vi "Array_extraction(SubVI).vi"(11 "Array":dbl[](array[numeric])) -> (1 "Value":dbl, 2 "Iteration":dbl, 3 "Info":dbl)   [LabVIEW 2017]
doc: "SubVI that extracts values from <B>Array</B> into three double values.\n<B>Info</B> - Contain information about what is in array(Velocity,RPM,Error etc.).\n<B>Value</B> - Contain value of read parameter.\n<B>Iteration</B> - Contain number of iteration in which data was read."
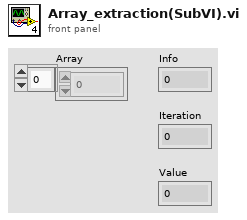
[diagram p1: front panel]
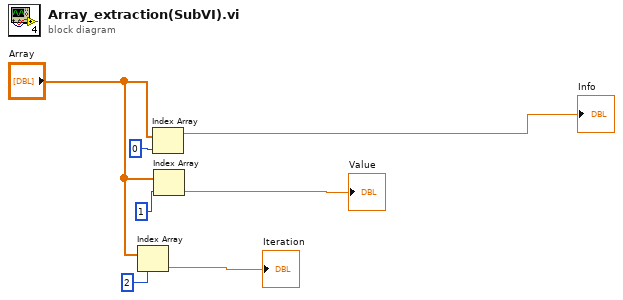
[diagram p0: block diagram]
diagram:
  n1 = Index Array(array="Array", index=2) -> (element=→"Iteration":dbl)
  n2 = Index Array(array="Array", index=0) -> (element=→"Info":dbl)
  n3 = Index Array(array="Array", index=1) -> (element=→"Value":dbl)
